vi "2 PulseMeasurements.vi"(2 "2 PulseMeas Chs":cluster{"DI0":refnum<k21>, "DI1":refnum<k21>}={"DI0"="NI 9411/DI0", "DI1"="NI 9411/DI1"}, 4 "PulseMeas Timeouts":u32[](array[numeric])=[0, 0]) -> (7 "PulseMeas Packets":u64[](array[numeric]))   [LabVIEW 2010]
uses:
  <vilib>/eio/EIONode/EIONode.xnode
  <vilib>/rvi/eio/nirviEIOImplementation/nirviEIOImplementation.xnode
  <vilib>/rvi/eio/common/nirviEmuClasses.ctl
  <vilib>/rvi/eio/common/nirviEmuTemplateMethod_noerrors.vi
  <vilib>/NI Veristand/FPGA/NI_VS FPGA Support.lvlib
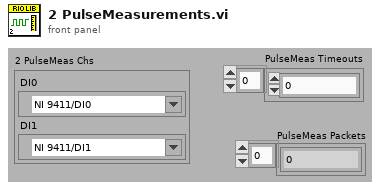
[diagram p1: front panel]
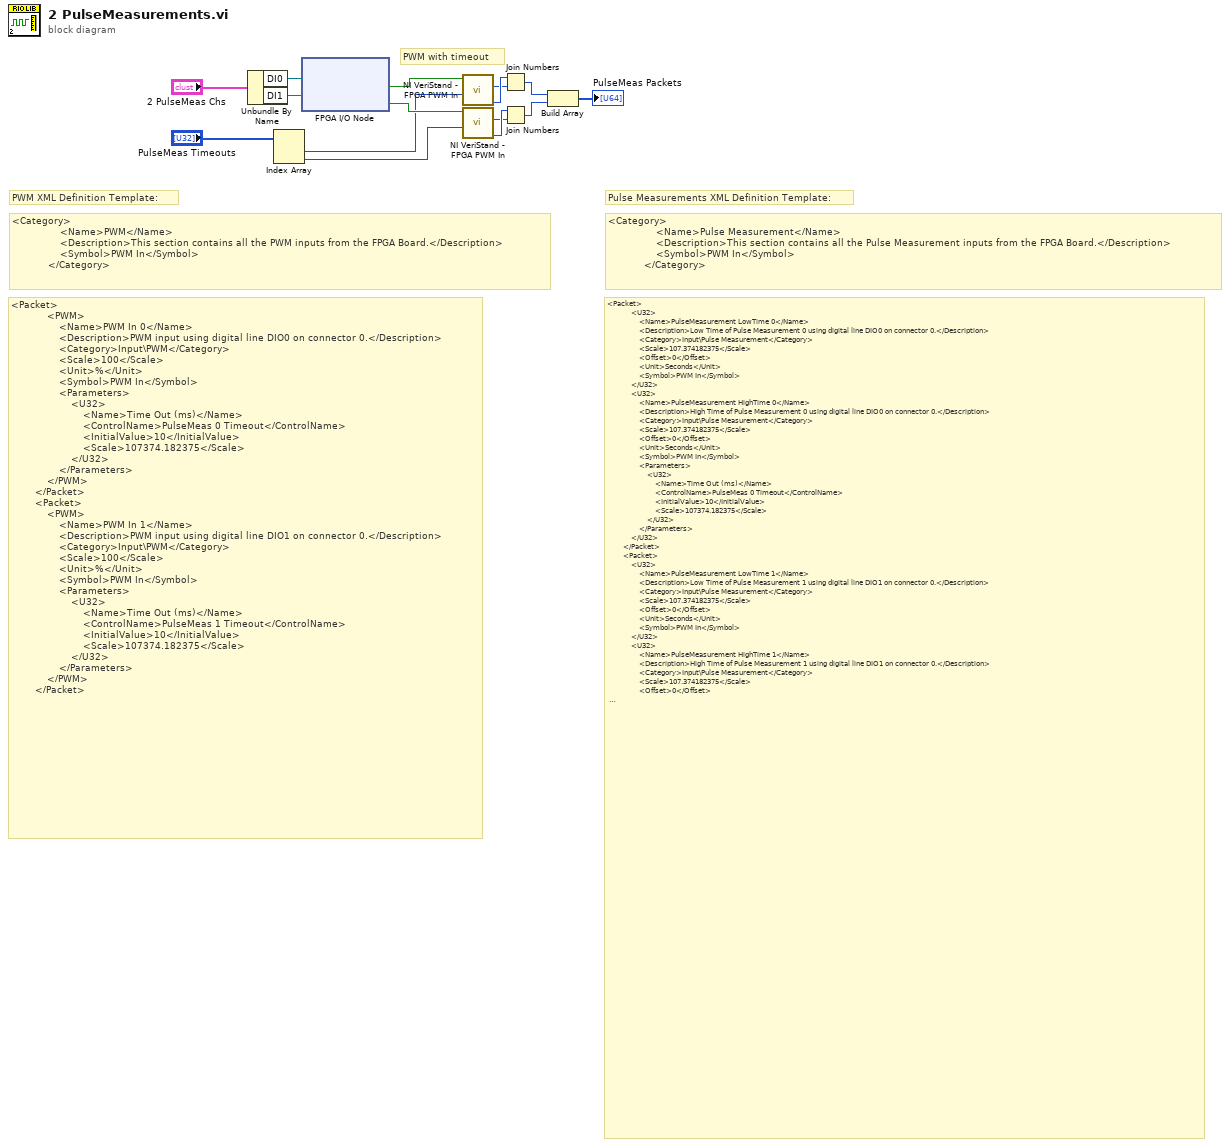
[diagram p0: block diagram]
diagram:
  # "<Category>\n                <Name>PWM</Name>\n                <Description>This section contains all the PWM inputs from the FPGA Board.</Description>\n                <Symbol>PWM In</Symbol>\n            </Category>"
  # "<Category>\n                <Name>Pulse Measurement</Name>\n                <Description>This section contains all the Pulse Measurement inputs from the FPGA Board.</Description>\n                <Symbol>PWM In</Symbol>\n            </Category>"
  # "Pulse Measurements XML Definition Template:"
  # "PWM XML Definition Template:"
  # "<Packet>\n            <PWM>\n                <Name>PWM In 0</Name>\n                <Description>PWM input using digital line DIO0 on connector 0.</Description>\n                <Category>Input\\PWM</Category>\n                <Scale>100</Scale>\n                <Unit>%</Unit>\n                <Symbol>PWM In</Symbol>\n                <Parameters>\n                    <U32>\n                        <Name>Time Out (ms)</Name>\n                        <ControlName>PulseMeas 0 Timeout</ControlName>\n                        <InitialValue>10</InitialValue>\n                        <Scale>107374.182375</Scale>\n                    </U32>\n                </Parameters>\n            </PWM>\n        </Packet>\n        <Packet>\n            <PWM>\n                <Name>PWM In 1</Name>\n                <Description>PWM input using digital line DIO1 on connector 0.</Description>\n                <Category>Input\\PWM</Category>\n                <Scale>100</Scale>\n                <Unit>%</Unit>\n                <Symbol>PWM In</Symbol>\n                <Parameters>\n                    <U32>\n                        <Name>Time Out (ms)</Name>\n                        <ControlName>PulseMeas 1 Timeout</ControlName>\n                        <InitialValue>10</InitialValue>\n                        <Scale>107374.182375</Scale>\n                    </U32>\n                </Parameters>\n            </PWM>\n        </Packet>"
  # "<Packet>\n            <U32>\n                <Name>PulseMeasurement LowTime 0</Name>\n                <Description>Low Time of Pulse Measurement 0 using digital line DIO0 on connector 0.</Description>\n                <Category>Input\\Pulse Measurement</Category>\n                <Scale>107.374182375</Scale>\n                <Offset>0</Offset>\n                <Unit>Seconds</Unit>\n                <Symbol>PWM In</Symbol>\n            </U32>\n            <U32>\n                <Name>PulseMeasurement HighTime 0</Name>\n                <Description>High Time of Pulse Measurement 0 using digital line DIO0 on connector 0.</Description>\n                <Category>Input\\Pulse Measurement</Category>\n                <Scale>107.374182375</Scale>\n                <Offset>0</Offset>\n                <Unit>Seconds</Unit>\n                <Symbol>PWM In</Symbol>\n                <Parameters>\n                    <U32>\n                        <Name>Time Out (ms)</Name>\n                        <ControlName>PulseMeas 0 Timeout</ControlName>\n                        <InitialValue>10</InitialValue>\n                        <Scale>107374.182375</Scale>\n                    </U32>\n                </Parameters>\n            </U32>\n        </Packet>\n        <Packet>\n            <U32>\n                <Name>PulseMeasurement LowTime 1</Name>\n                <Description>Low Time of Pulse Measurement 1 using digital line DIO1 on connector 0.</Description>\n                <Category>Input\\Pulse Measurement</Category>\n                <Scale>107.374182375</Scale>\n                <Offset>0</Offset>\n                <Unit>Seconds</Unit>\n                <Symbol>PWM In</Symbol>\n            </U32>\n            <U32>\n                <Name>PulseMeasurement HighTime 1</Name>\n                <Description>High Time of Pulse Measurement 1 using digital line DIO1 on connector 0.</Description>\n                <Category>Input\\Pulse Measurement</Category>\n                <Scale>107.374182375</Scale>\n                <Offset>0</Offset>\n                <Unit>Seconds</Unit>\n                <Symbol>PWM In</Symbol>\n                <Parameters>\n                    <U32>\n                        <Name>Time Out (ms)</Name>\n                        <ControlName>PulseMeas 1 Timeout</ControlName>\n                        <InitialValue>10</InitialValue>\n                        <Scale>107374.182375</Scale>\n                    </U32>\n                </Parameters>\n            </U32>\n        </Packet>"
  # "PWM with timeout"
  n1 = Unbundle By Name("2 PulseMeas Chs") -> ("DI0"=w1:refnum<k21>, "DI1"=w2:refnum<k21>)
  n2 = Index Array(array="PulseMeas Timeouts") -> (element #1=w4:u32, element #2=w5:u32)  [unwired: 2 in]
  n3 = xnode "FPGA I/O Node"("FPGA I/O In"=w1, "FPGA I/O In"=w2) -> ("I/O Item"=w7:bool, "I/O Item"=w10:bool)  [unwired: 2 out]
  n4 = call <vilib>:"NI VeriStand - FPGA PWM In.vi"("Time Out"=w4, "Value"=w7) -> ("High time"=w9:u32, "Low Time"=w8:u32)  [unwired: 8 out]
  n5 = call <vilib>:"NI VeriStand - FPGA PWM In.vi"("Time Out"=w5, "Value"=w10) -> ("High time"=w12:u32, "Low Time"=w11:u32)  [unwired: 8 out]
  n6 = Join Numbers(hi=w9, lo=w8) -> ((hi.lo)=w13:u64)
  n7 = Join Numbers(hi=w12, lo=w11) -> ((hi.lo)=w14:u64)
  n8 = Build Array(w13, w14) -> (→"PulseMeas Packets":u64[])
